vi "Compare ECAT Vars.vi"(8 "Fehler (Eingang, kein Fehler)":errorcluster, 11 "I/O Output Vars (Eingang)":T1[](array[typedef]) {"VS ref" format="%.0x"}) -> (0 "Fehler (Ausgang)":errorcluster, 3 "I/O Output Vars (Ausgang)":T1[](array[typedef]) {"VS ref" format="%.0x"})   [LabVIEW 2017, in "Scan Engine Custom Device.lvlib"]
uses:
  Scan Engine Custom Device.lvlib
  Type Defs/Generic ECAT Slave IOV Cluster.ctl
  <vilib>/NI Veristand/Custom Device API/Custom Device Item Ref.ctl
  Type Defs/UDV Data Type.ctl
  Globals/Property Strings.vi
  <vilib>/NI Veristand/Custom Device API/Get Item Property (String).vi
  <vilib>/NI Veristand/Custom Device API/Get Item Property (I32).vi
  Globals/Error Strings.vi
  <vilib>/NI VeriStand/Custom Device API/Custom Device API.lvlib
  <vilib>/NI Veristand/Custom Device Tools/Custom Device Utility Library/Custom Device Utility Library.lvlib
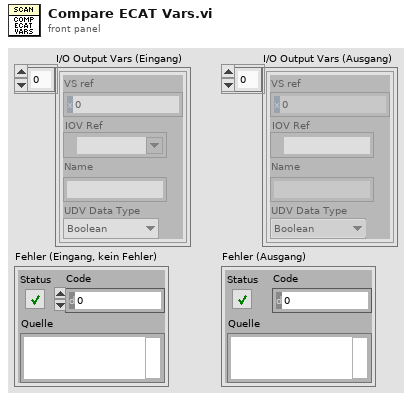
[diagram p1: front panel]
types:
  T1 = typedef "Scan Engine Custom Device.lvlib/Generic ECAT Slave IOV Cluster.ctl" = cluster{"VS ref":T2, "IOV Ref":refnum<k21>, "Name":string, "UDV Data Type":T3}
  T2 = typedef "Custom Device API.lvlib/Custom Device Item Ref.ctl" = u64
  T3 = typedef "Scan Engine Custom Device.lvlib/UDV Data Type.ctl" = enum16{"Boolean", "Fixed Point", "Int8", "Int16", "Int32", "Int64", "U32 Bit Field", "UInt8", "UInt16", "UInt32", "UInt64", "Other"}
  T4 = typedef "Custom Device API.lvlib/Custom Device Item Info.ctl" = cluster{"Name":string, "Is Channel":bool, "GUID":string, "Is Waveform":bool}
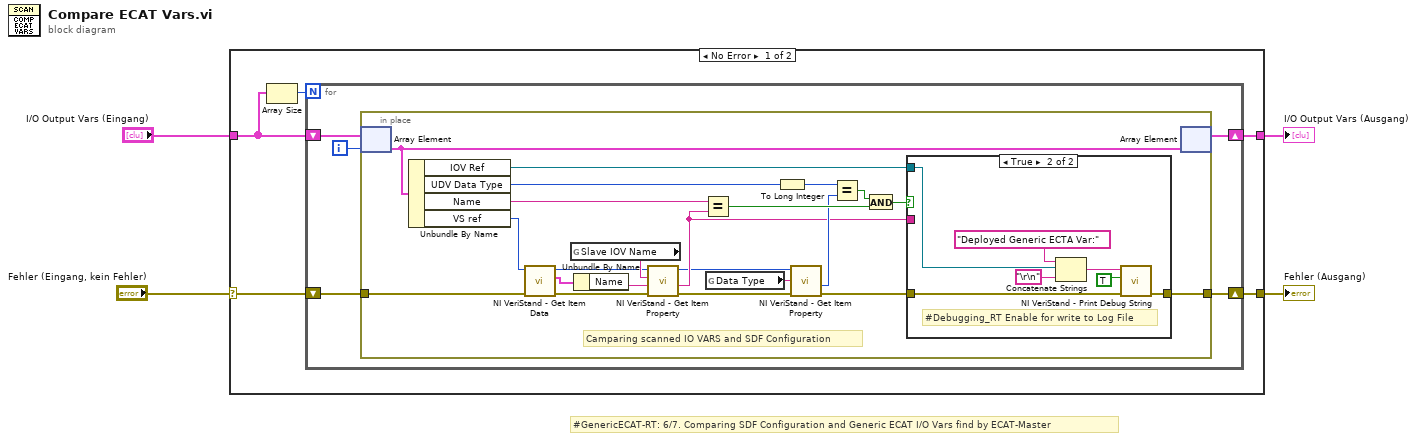
[diagram p0: block diagram]
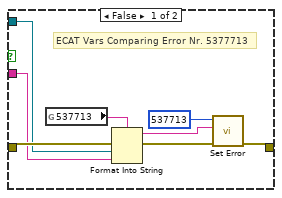
[diagram p2: hidden frame]
diagram:
  # "#GenericECAT-RT: 6/7. Comparing SDF Configuration and Generic ECAT I/O Vars find by ECAT-Master"
  n1 = case shown="No Error" "Fehler (Eingang, kein Fehler)" {
    selector: "Fehler (Eingang, kein Fehler)" -> [w6 w52]
    tunnel: [w9 w53] -> w4
    tunnel: [w5 w52] -> w3
    tunnel: "I/O Output Vars (Eingang)" -> [w8 w53]
    frame No Error {
      n2 = Array Size(array=w8) -> (size(s)=w7:i32)
      n3 = for {
        N: w7 -> [_]
        shift-right: [w10] -> w5
        shift-left: w6 -> [w12]
        shift-right: [w11] -> w9
        shift-left: w8 -> [w14]
        i -> [w13]
        n4 = in-place {
          in-place-border: w12 -> [w19]
          in-place-border: [w30] -> w10
          # "Camparing scanned IO VARS and SDF Configuration"
          n5 = in-place-array #1(w14, w13) -> (w35:T1)
          n6 = Unbundle By Name(w35) -> ("IOV Ref"=w25:refnum<k21>, "UDV Data Type"=w27:T3, "Name"=w29:string, "VS ref"=w20:T2)
          n7 = call <vilib>:"NI VeriStand - Get Item Data.vi"("error in (no error)"=w19, "Item Ref in"=w20) -> ("error out"=w24:errorcluster, "Item Info"=w21:T4, "Item Ref out"=w16:T2)  [unwired: 6 in, 1 out]
          n8 = global read "Property Strings.vi" "Slave IOV Name"() -> (w22:string)
          n9 = Unbundle By Name(w21) -> ("Name"=w23:string)
          n10 = call-poly <vilib>:"NI VeriStand - Get Item Property.vi"("error in (no error)"=w24, "Default Value"=w23, "Property Name"=w22, "Item Ref in"=w16) -> ("error out"=w18:errorcluster, "Value"=w17:string, "Item Ref out"=w15:T2)  [unwired: 4 in, 1 out]
          n11 = Equal?(x=w29, y=w17) -> (x = y?=w33:bool)
          n12 = global read "Property Strings.vi" "Data Type"() -> (w36:string)
          n13 = To Long Integer(number=w27) -> (32bit integer=w26:i32)
          n14 = call-poly <vilib>:"NI VeriStand - Get Item Property.vi"("error in (no error)"=w18, "Property Name"=w36, "Item Ref in"=w15) -> ("error out"=w31:errorcluster, "Value"=w28:i32)  [unwired: 5 in, 2 out]
          n15 = Equal?(x=w26, y=w28) -> (x = y?=w34:bool)
          n16 = And(x=w34, y=w33) -> (x .and. y?=w32:bool)
          n17 = case shown="True" w32 {
            tunnel: w31 -> [w40 w51]
            tunnel: [w39 w50] -> w30
            tunnel: w25 -> [w38 w46]
            tunnel: w17 -> [w37 _]
            frame False {
              # "ECAT Vars Comparing Error Nr. 5377713"
              n18 = global read "Error Strings.vi" "537713"() -> (w41:string)
              n19 = Format Into String(format string=w41, error in=w40, w38, w37) -> (resulting string=w43:string, error out=w42:errorcluster)  [unwired: 1 in]
              n20 = call "Set Error.vi"("error in (no error)"=w42, "Message"=w43, "Code"=537713 ("error code (0)")) -> ("error out"=w39:errorcluster)  [unwired: 8 in]
            }
            frame True {
              # "#Debugging_RT Enable for write to Log File"
              n21 = Concatenate Strings("Deployed Generic ECTA Var:", w46, "\r\n") -> (w49:string)
              n22 = call <vilib>:"NI VeriStand - Print Debug String.vi"("error in (no error)"=w51, "Add to log file? (T)"=TRUE, "Message"=w49) -> ("error out"=w50:errorcluster)  [unwired: 8 in]
            }
          }
          n23 = in-place-array #1(w35) -> (w11:T1[])  [unwired: 1 out]
        }
      }
    }
    frame Error {
    }
  }
  "I/O Output Vars (Ausgang)" <- w4
  "Fehler (Ausgang)" <- w3
